vi "Check Downcast (Multiple).vi"(8 "error in (no error)":errorcluster, 11 "xceDataNode In":refnum<class "xceDataNode.lvclass">) -> (0 "error out":errorcluster, 1 "Ok?":bool, 3 "xceDataNode Out":refnum<class "xceDataNode.lvclass">)   [LabVIEW 2013, in "FPGADMAChannelData.lvclass"]
uses:
  FPGADMAChannelData.lvclass
  xCE/xceDataNode/xceDataNode.lvclass
  DMA_Read/DMA_Read.lvclass
  DMA_Write/DMA_Write.lvclass
  Packet/Packet.lvclass
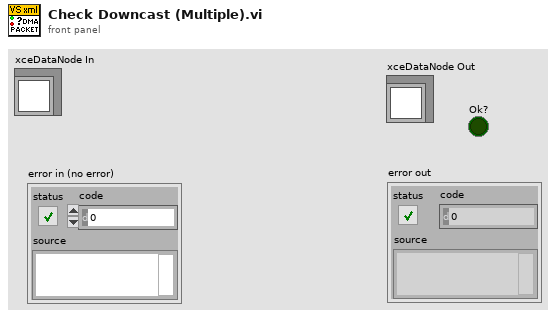
[diagram p1: front panel]
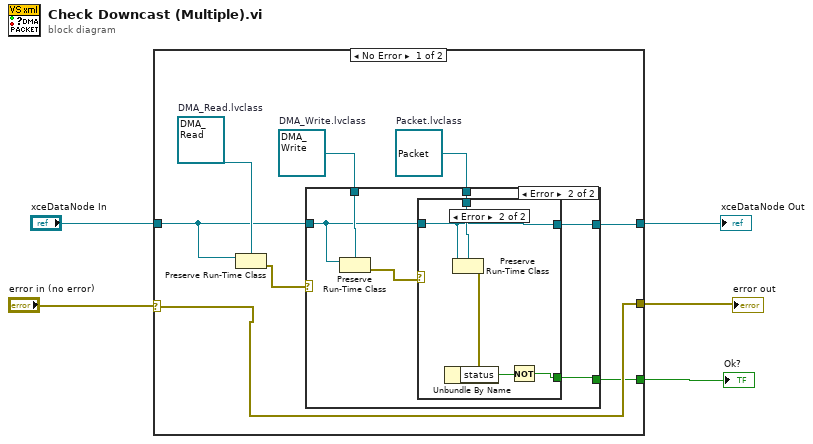
[diagram p0: block diagram]
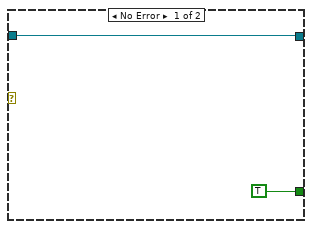
[diagram p2: hidden frame]
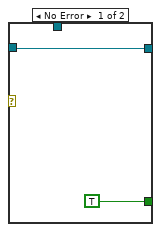
[diagram p3: hidden frame]
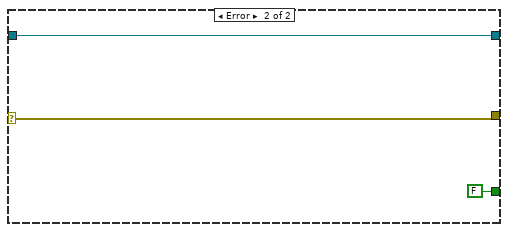
[diagram p4: hidden frame]
diagram:
  n1 = case shown="No Error" "error in (no error)" {
    selector: "error in (no error)" -> [w8 w30]
    tunnel: "xceDataNode In" -> [w6 w31]
    tunnel: [w10 w31] -> w4
    tunnel: [w8 w30] -> w2
    tunnel: [w7 FALSE] -> w1
    frame No Error {
      w9 = refnum<class "Packet.lvclass"> refnum  # Packet.lvclass
      w11 = refnum<class "DMA_Write.lvclass"> refnum  # DMA_Write.lvclass
      w13 = refnum<class "DMA_Read.lvclass"> refnum  # DMA_Read.lvclass
      n2 = Preserve Run-Time Class(object in=w6, 2:w13) -> (error out=w12:errorcluster)  [unwired: 1 in, 1 out]
      n3 = case shown="Error" w12 {
        tunnel: w6 -> [w15 w16]
        tunnel: w11 -> [_ w21]
        tunnel: [w15 w19] -> w10
        tunnel: w9 -> [_ w18]
        tunnel: [TRUE w17] -> w7
        frame No Error {
        }
        frame Error {
          n4 = Preserve Run-Time Class(object in=w16, 2:w21) -> (error out=w20:errorcluster)  [unwired: 1 in, 1 out]
          n5 = case shown="Error" w20 {
            tunnel: w16 -> [w23 w24]
            tunnel: [w23 w24] -> w19
            tunnel: w18 -> [_ w28]
            tunnel: [TRUE w25] -> w17
            frame No Error {
            }
            frame Error {
              n6 = Preserve Run-Time Class(object in=w24, 2:w28) -> (error out=w27:errorcluster)  [unwired: 1 in, 1 out]
              n7 = Unbundle By Name(w27) -> ("status"=w26:bool)
              n8 = Not(x=w26) -> (.not. x?=w25:bool)
            }
          }
        }
      }
    }
    frame Error {
    }
  }
  "xceDataNode Out" <- w4
  "error out" <- w2
  "Ok?" <- w1
